vi "Add Width and Height to Bounds.vi"(1 "WinBounds":T1) -> (0 "Bounds Out":T2)   [LabVIEW 2020]
uses:
  <vilib>/Utility/miscctls.llb/LVRectTypeDef.ctl
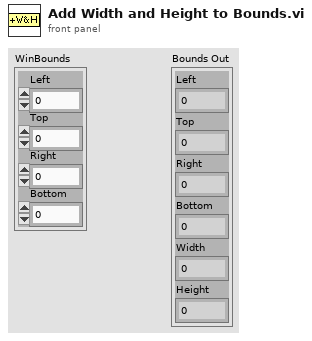
[diagram p1: front panel]
types:
  T1 = typedef "LVRectTypeDef.ctl" = cluster{"Left":i16, "Top":i16, "Right":i16, "Bottom":i16}
  T2 = cluster{"Left":i16, "Top":i16, "Right":i16, "Bottom":i16, "Width":i16, "Height":i16}
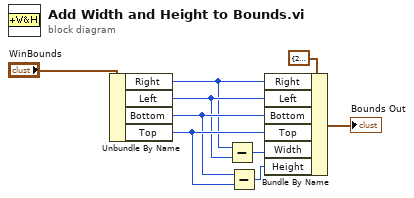
[diagram p0: block diagram]
diagram:
  n1 = Unbundle By Name("WinBounds") -> ("Right"=w4:i16, "Left"=w5:i16, "Bottom"=w7:i16, "Top"=w8:i16)
  n2 = Subtract(x=w4, y=w5) -> (x-y=w6:i16)
  n3 = Subtract(x=w7, y=w8) -> (x-y=w9:i16)
  n4 = Bundle By Name(cluster=T2 {"Left"=2317, "Top"=194, "Right"=3443, "Bottom"=1006, "Width"=1006, "Height"=3443} ("Front Panel Window:Window Bounds 2"), "Right"=w4, "Left"=w5, "Bottom"=w7, "Top"=w8, "Width"=w6, "Height"=w9) -> (→"Bounds Out":T2)
